vi "testMinDistanceToObstaclewAng.vi"() -> ()   [LabVIEW 2013]
uses:
  Data/TypeDefs/UTM Location.ctl
  Obstacle.lvclass
panel:
  out "Closest point to boat":T1 {"North" format="%#_10f"; "East" format="%#_8f"}
  out "Min angle (deg)":dbl
  out "Min angle (rad)":dbl
  out "Min distance":dbl
  in  "Boat":T1={"UTM Zone"=0.0, "Hemisphere"=enum."North", "East"=10.0, "North"=0.0} {"North" format="%#_10f"; "East" format="%#_8f"}
  in  "Input List of UTM locations to be arranged into segments":T1[](array[typedef])=[{"UTM Zone"=0.0, "Hemisphere"=enum."North", "East"=0.0, "North"=0.0}, {"UTM Zone"=0.0, "Hemisphere"=enum."North", "East"=5.0, "North"=0.0}, {"UTM Zone"=0.0, "Hemisphere"=enum."North", "East"=0.0, "North"=5.0}, {"UTM Zone"=0.0, "Hemisphere"=enum."North", "East"=-5.0, "North"=0.0}] {"North" format="%#_10f"; "East" format="%#_8f"}
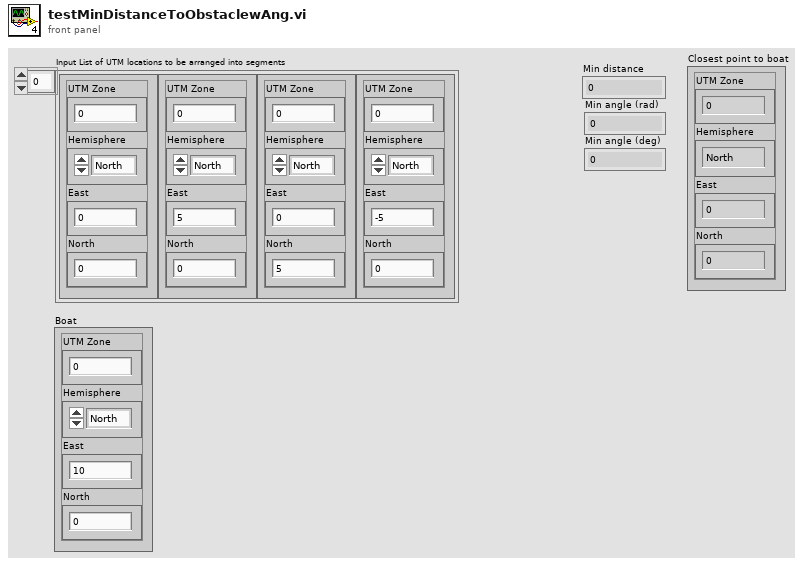
[diagram p1: front panel]
types:
  T1 = typedef "UTM Location.ctl" = cluster{"UTM Zone":dbl, "Hemisphere":enum16{"North", "South"}, "East":dbl, "North":dbl}
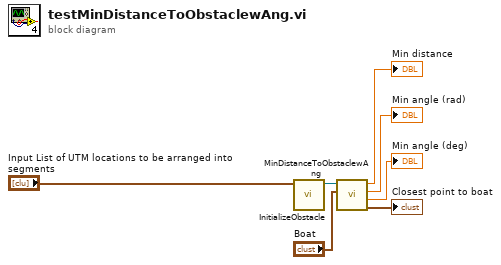
[diagram p0: block diagram]
diagram:
  n1 = call "InitializeObstacle.vi"("Input List of UTM locations to be arranged into segments"="Input List of UTM locations to be arranged into segments") -> ("Obstacle.lvclass"=w6:refnum<class "Obstacle.lvclass">)  [unwired: 10 in]
  n2 = call "MinDistanceToObstaclewAng.vi"("Boat"="Boat", "Obstacle.lvclass"=w6) -> ("Closest point to boat"=→"Closest point to boat":T1, "Min angle (deg)"=→"Min angle (deg)":dbl, "Min angle (rad)"=→"Min angle (rad)":dbl, "Min distance"=→"Min distance":dbl)  [unwired: 6 in]
